vi "Veronica Maria - Simulador do Computador de Bordo.vi"() -> ()   [LabVIEW 2015]
uses:
  <vilib>/Instr/_visa.llb/VISA Configure Serial Port (Instr).vi
panel:
  out "Gráfico 2":u8(graph)
  out "Erro no diretório 2":errorcluster
  out "Arquivo Hexadecimal":refnum<file>
  out "Tempo da Varredura":dbl
  in  "DATA SEND":bool
  in  "DATA SEND":bool
  out "Erro serial":errorcluster
  out "Bytes Recebidos":u16
  out "Botao Selecionado":string
  out "Erros de entrada":errorcluster
  out "Erro no diretório":errorcluster
  out "Arquivo":refnum<file>
  out "Erros de envio entrada":errorcluster
  out "Saída de VISA Resource Name":refnum<visa-resource-name>
  out "PACOTE RECEBIDO":string
  out "frames":u8[][](array[numeric])
  out "frame enviado":u8[](array[numeric]) format="%x"
  in  "TURN OFF":bool
  in  "TURN ON":bool
  in  "DESLIGAR":bool
  in  "RESET":bool
  in  "DATA REQUEST":bool
  in  "diretório do arquivo":string="C:\\Testes\\"
  in  "bits de parada (8: 1 bit)":u8(ring)=10 items=["2.0"=20, "1.5"=15, "1.0"=10]
  in  "controle de fluxo (0: none)":u8(ring) items=["None", "XON/XOFF", "RTS/CTS", "XON/XOFF & RTS/CTS", "DTR/DSR", "XON/XOFF & DTS/DSR"]
  in  "taxa de transmissão (9600)":u16=9600
  in  "paridade (0: none)":u8(ring) items=["None", "Odd", "Even", "Mark", "Space"]
  in  "porta":refnum<visa-resource-name>
  in  "bits de dados(8)":u8=8 min=5 max=8 step=1
  # "Configurações \ndo \nSistema"
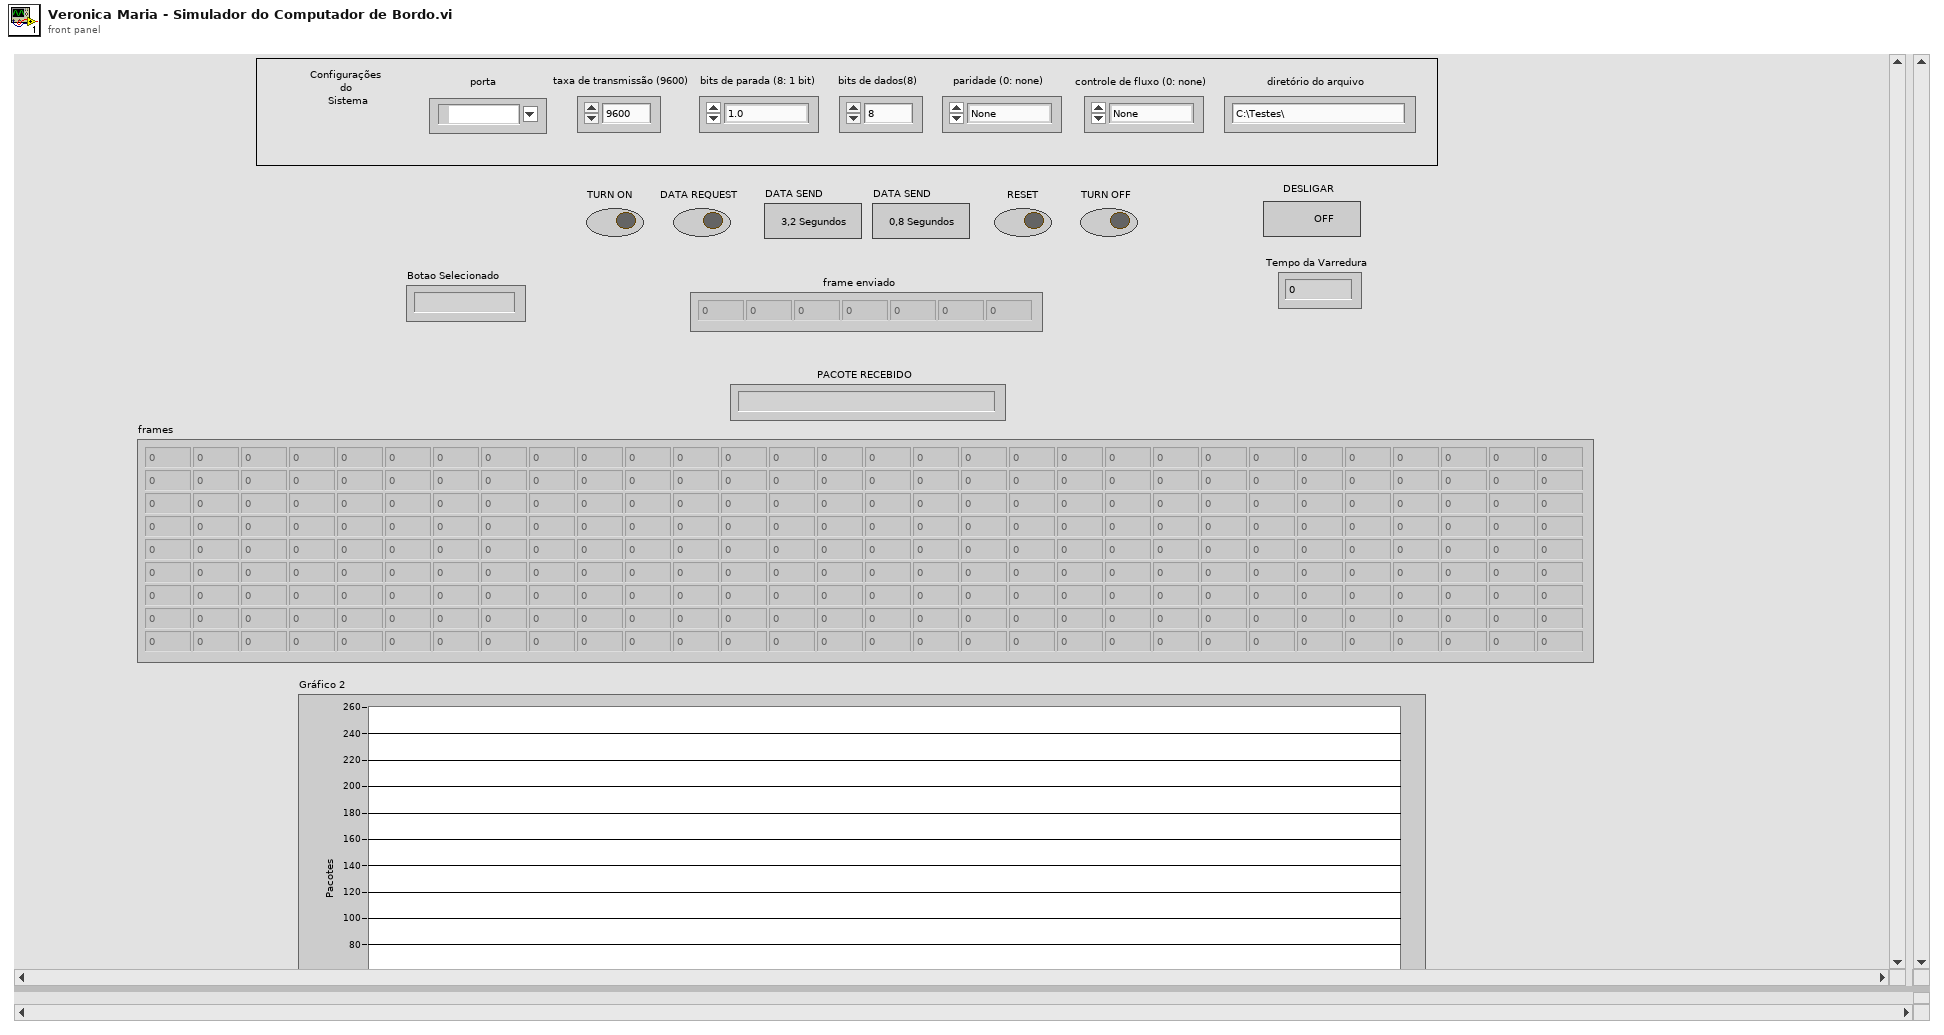
[diagram p1: front panel]
types:
  T1 = enum16{"open", "replace", "create", "open or create", "replace or create", "replace or create with confirmation"}
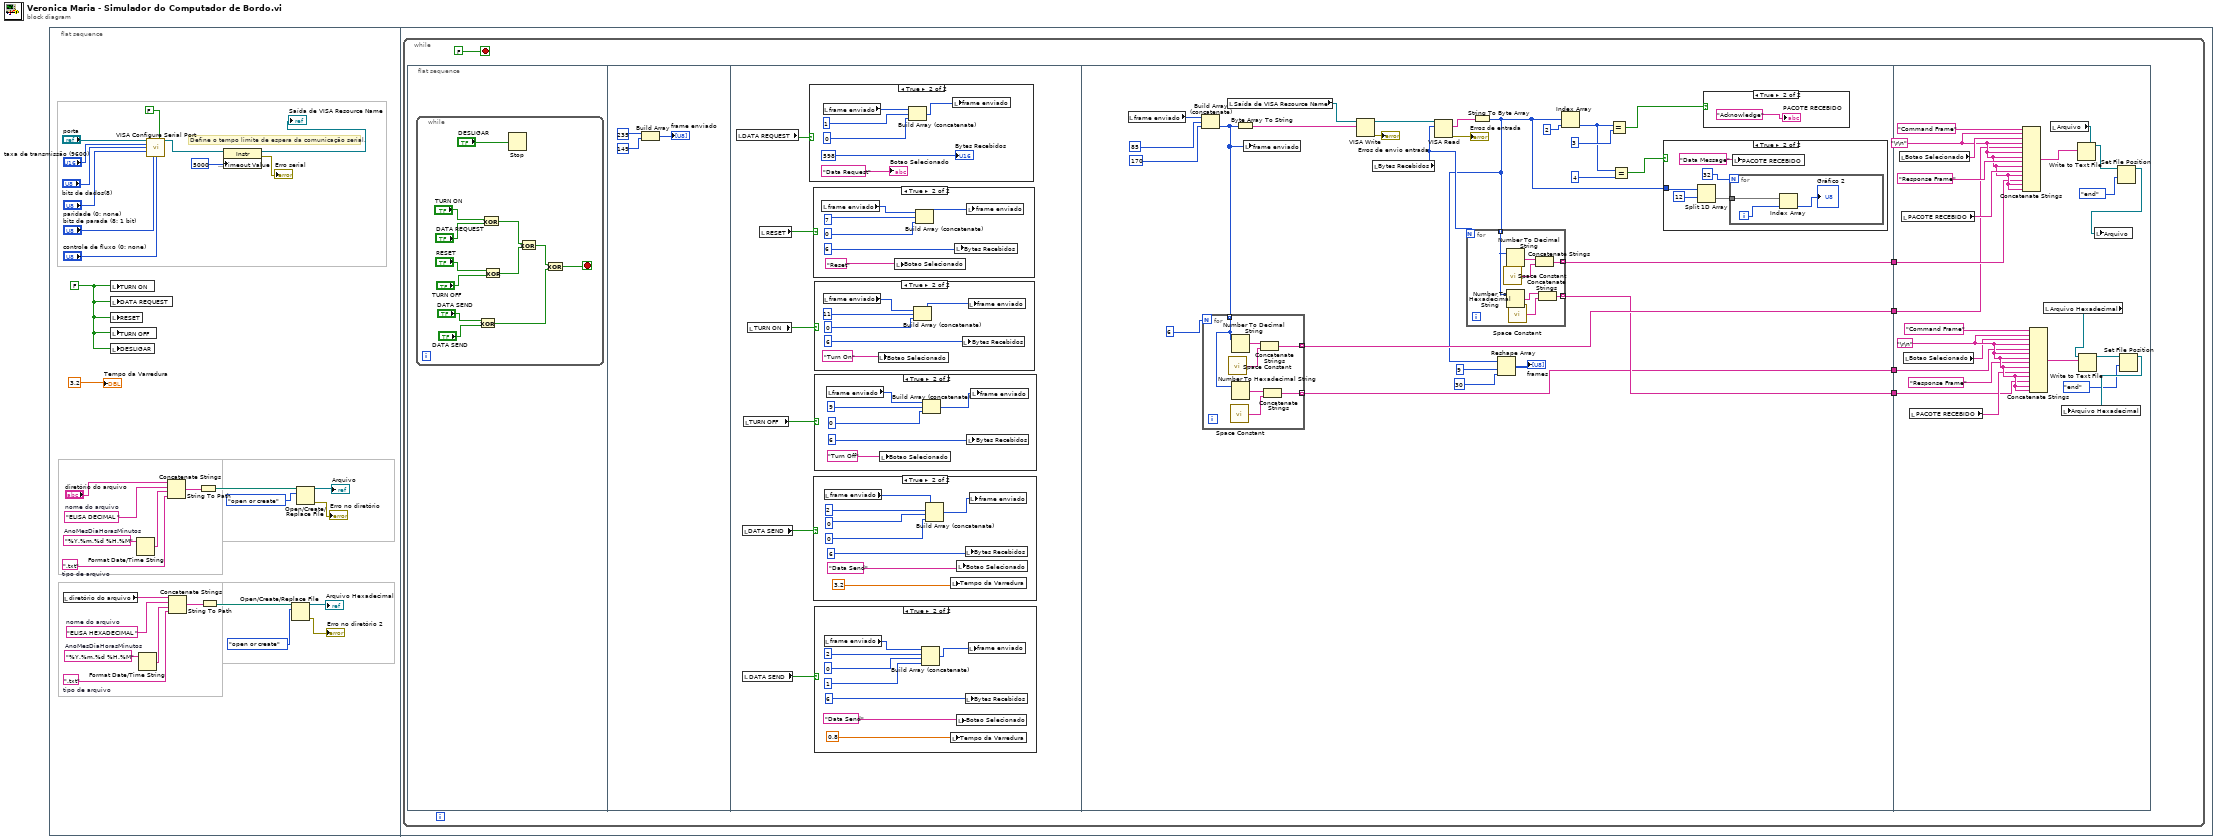
[diagram p0: block diagram]
diagram:
  n1 = flat-sequence {
    frame #0 {
      w10 = "%Y.%m.%d %H.%M"  # AnoMesDiaHorasMinutos
      w7 = ".txt"  # tipo de arquivo
      w9 = "ELISA HEXADECIMAL "  # nome do arquivo
      w16 = FALSE
      w26 = "%Y.%m.%d %H.%M"  # AnoMesDiaHorasMinutos
      w23 = ".txt"  # tipo de arquivo
      w25 = "ELISA DECIMAL "  # nome do arquivo
      # "Define o tempo limite de espera da comunicação serial."
      n2 = local read "diretório do arquivo"() -> (w1:string)
      n3 = local write "TURN ON"(w16) -> ()
      n4 = local write "DATA REQUEST"(w16) -> ()
      n5 = local write "RESET"(w16) -> ()
      n6 = local write "TURN OFF"(w16) -> ()
      n7 = local write "DESLIGAR"(w16) -> ()
      n8 = Format Date/Time String(time format string (%c)=w26) -> (date/time string=w24:string)  [unwired: 2 in]
      n9 = Format Date/Time String(time format string (%c)=w10) -> (date/time string=w8:string)  [unwired: 2 in]
      n10 = call-poly "VISA Configure Serial Port"("VISA resource name"="porta", "Enable Termination\nChar (T)"=FALSE, "baud rate (9600)"="taxa de transmissão (9600)", "data bits (8)"="bits de dados(8)", "parity (0:none)"="paridade (0: none)", "stop bits (10: 1 bit)"="bits de parada (8: 1 bit)", "flow control (0:none)"="controle de fluxo (0: none)") -> ("VISA resource name out"=w13:refnum<visa-resource-name>)  [unwired: 7 in, 1 out]
      n11 = Concatenate Strings("diretório do arquivo", w25, w24, w23) -> (w22:string)
      n12 = Concatenate Strings(w1, w9, w8, w7) -> (w6:string)
      n13 = String To Path(string=w22) -> (path=w21:path)
      n14 = String To Path(string=w6) -> (path=w3:path)
      n15 = property class="Instr"(reference=w13, "General Settings:Timeout Value"=u32 5000) -> (reference out=→"Saída de VISA Resource Name":refnum<visa-resource-name>, error out=→"Erro serial":errorcluster)  [unwired: 1 in]
      n16 = Open/Create/Replace File(file path (use dialog)=w3, operation (0:open)=T1."open or create") -> (refnum out=→"Arquivo Hexadecimal":refnum<file>, error out=→"Erro no diretório 2":errorcluster)  [unwired: 4 in, 1 out]
      n17 = Open/Create/Replace File(file path (use dialog)=w21, operation (0:open)=T1."open or create") -> (refnum out=→"Arquivo":refnum<file>, error out=→"Erro no diretório":errorcluster)  [unwired: 4 in, 1 out]
      "Tempo da Varredura" <- 3.2
    }
    frame #1 {
      n18 = while {
        stop <- FALSE stop-if-true
        n19 = flat-sequence {
          tunnel: [w109] -> w37
          tunnel: [w108] -> w36
          tunnel: [w100] -> w35
          tunnel: [w101] -> w34
          tunnel: w37 -> [w162]
          tunnel: w36 -> [w161]
          tunnel: w35 -> [w155]
          tunnel: w34 -> [w154]
          frame #0 {
            n20 = while {
              stop <- w39 stop-if-true
              n21 = Exclusive Or(1:"DATA SEND", 2:"DATA SEND") -> (0:w40:bool)
              n22 = Exclusive Or(1:"DATA REQUEST", 2:"TURN ON") -> (0:w43:bool)
              n23 = Exclusive Or(1:"TURN OFF", 2:"RESET") -> (0:w42:bool)
              n24 = Stop(stop? (T)="DESLIGAR") -> ()
              n25 = Exclusive Or(1:w42, 2:w43) -> (0:w41:bool)
              n26 = Exclusive Or(1:w40, 2:w41) -> (0:w39:bool)
            }
          }
          frame #1 {
            n27 = Build Array(235, 149) -> (→"frame enviado":i32[])
          }
          frame #2 {
            n28 = local read "DATA REQUEST"() -> (w59:bool)
            n29 = local read "DATA SEND"() -> (w55:bool)
            n30 = local read "DATA SEND"() -> (w54:bool)
            n31 = local read "TURN OFF"() -> (w56:bool)
            n32 = local read "TURN ON"() -> (w57:bool)
            n33 = local read "RESET"() -> (w58:bool)
            n34 = case shown="True" w59 {
              frame False {
              }
              frame True {
                n35 = local read "frame enviado"() -> (w99:u8[])
                n36 = Build Array (concatenate)(w99, 1, 0) -> (w95:i32[])
                n37 = local write "frame enviado"(w95) -> ()
                "Botao Selecionado" <- "Data Request"
                "Bytes Recebidos" <- 598
              }
            }
            n38 = case shown="True" w58 {
              frame False {
              }
              frame True {
                n39 = local read "frame enviado"() -> (w93:u8[])
                n40 = local write "Botao Selecionado"("Reset") -> ()
                n41 = Build Array (concatenate)(w93, 7, 0) -> (w90:i32[])
                n42 = local write "Bytes Recebidos"(6) -> ()
                n43 = local write "frame enviado"(w90) -> ()
              }
            }
            n44 = case shown="True" w55 {
              frame False {
              }
              frame True {
                n45 = local read "frame enviado"() -> (w75:u8[])
                n46 = Build Array (concatenate)(w75, 2, 0, 0) -> (w73:i32[])
                n47 = local write "Tempo da Varredura"(3.2) -> ()
                n48 = local write "Botao Selecionado"("Data Send") -> ()
                n49 = local write "Bytes Recebidos"(6) -> ()
                n50 = local write "frame enviado"(w73) -> ()
              }
            }
            n51 = case shown="True" w57 {
              frame False {
              }
              frame True {
                n52 = local read "frame enviado"() -> (w87:u8[])
                n53 = local write "Botao Selecionado"("Turn On") -> ()
                n54 = Build Array (concatenate)(w87, 11, 0) -> (w84:i32[])
                n55 = local write "Bytes Recebidos"(6) -> ()
                n56 = local write "frame enviado"(w84) -> ()
              }
            }
            n57 = case shown="True" w56 {
              frame False {
              }
              frame True {
                n58 = local read "frame enviado"() -> (w80:u8[])
                n59 = local write "Botao Selecionado"("Turn Off") -> ()
                n60 = Build Array (concatenate)(w80, 9, 0) -> (w78:i32[])
                n61 = local write "Bytes Recebidos"(6) -> ()
                n62 = local write "frame enviado"(w78) -> ()
              }
            }
            n63 = case shown="True" w54 {
              frame False {
              }
              frame True {
                n64 = local read "frame enviado"() -> (w67:u8[])
                n65 = Build Array (concatenate)(w67, 2, 0, 1) -> (w66:i32[])
                n66 = local write "Tempo da Varredura"(0.8) -> ()
                n67 = local write "Botao Selecionado"("Data Send") -> ()
                n68 = local write "Bytes Recebidos"(6) -> ()
                n69 = local write "frame enviado"(w66) -> ()
              }
            }
          }
          frame #3 {
            n70 = local read "frame enviado"() -> (w125:u8[])
            n71 = Build Array (concatenate)(w125, 85, 170) -> (w123:i32[])
            n72 = for {
              N: 6 -> [_]
              tunnel: w123 -> [w145] mode=indexing
              tunnel: [w147] -> w108 mode=indexing
              tunnel: [w142] -> w100 mode=indexing
              n73 = call <vilib>:"Space Constant.vi"() -> ("String"=w148:string)
              n74 = call <vilib>:"Space Constant.vi"() -> ("String"=w143:string)
              n75 = Number To Decimal String(number=w145) -> (decimal integer string=w146:string)  [unwired: 1 in]
              n76 = Number To Hexadecimal String(2:w145) -> (0:w144:string)  [unwired: 1 in]
              n77 = Concatenate Strings(w146, w148) -> (w147:string)
              n78 = Concatenate Strings(w144, w143) -> (w142:string)
            }
            n79 = local read "Saída de VISA Resource Name"() -> (w121:refnum<visa-resource-name>)
            n80 = Byte Array To String(unsigned byte array=w123) -> (string=w122:string)
            n81 = local write "frame enviado"(w123) -> ()
            n82 = VISA Write(VISA resource name=w121, write buffer=w122) -> (VISA resource name out=w119:refnum<visa-resource-name>, error out=→"Erros de envio entrada":errorcluster)  [unwired: 1 in, 1 out]
            n83 = local read "Bytes Recebidos"() -> (w110:u16)
            n84 = VISA Read(VISA resource name=w119, byte count=w110) -> (read buffer=w117:string, error out=→"Erros de entrada":errorcluster)  [unwired: 1 in, 2 out]
            n85 = String To Byte Array(string=w117) -> (unsigned byte array=w102:u8[])
            n86 = for {
              N: w110 -> [_]
              tunnel: w102 -> [w136] mode=indexing
              tunnel: [w140] -> w109 mode=indexing
              tunnel: [w135] -> w101 mode=indexing
              n87 = call <vilib>:"Space Constant.vi"() -> ("String"=w141:string)
              n88 = Number To Decimal String(number=w136) -> (decimal integer string=w139:string)  [unwired: 1 in]
              n89 = Number To Hexadecimal String(2:w136) -> (0:w138:string)  [unwired: 1 in]
              n90 = call <vilib>:"Space Constant.vi"() -> ("String"=w137:string)
              n91 = Concatenate Strings(w139, w141) -> (w140:string)
              n92 = Concatenate Strings(w138, w137) -> (w135:string)
            }
            n93 = Reshape Array(w102, u8 9, u8 30) -> (→"frames":u8[][])
            n94 = Index Array(array=w102, index=u8 2) -> (element=w107:u8)
            n95 = Equal?(x=w107, y=u8 3 ("index")) -> (x = y?=w111:bool)
            n96 = Equal?(x=w107, y=u8 4 ("index")) -> (x = y?=w105:bool)
            n97 = case shown="True" w105 {
              tunnel: w102 -> [_ w127]
              frame False {
              }
              frame True {
                n98 = Split 1D Array(array=w127, index=u8 12) -> (second subarray=w128:u8[])  [unwired: 1 out]
                n99 = for {
                  N: 32 -> [_]
                  tunnel: w128 -> [w133]
                  i -> [w132]
                  n100 = Index Array(array=w133, index=w132) -> (element=→"Gráfico 2":u8)
                }
                n101 = local write "PACOTE RECEBIDO"("Data Message") -> ()
              }
            }
            n102 = case shown="True" w111 {
              frame False {
              }
              frame True {
                "PACOTE RECEBIDO" <- "Acknowledge"
              }
            }
          }
          frame #4 {
            w159 = "\r\n"
            w163 = "\r\n"
            n103 = local read "Botao Selecionado"() -> (w166:string)
            n104 = local read "PACOTE RECEBIDO"() -> (w164:string)
            n105 = local read "Botao Selecionado"() -> (w158:string)
            n106 = local read "PACOTE RECEBIDO"() -> (w156:string)
            n107 = Concatenate Strings("Command Frame", w163, w166, w163, w161, w163, w163, "Response Frame", w163, w164, w163, w162, w163, w163) -> (w171:string)
            n108 = Concatenate Strings("Command Frame", w159, w158, w159, w155, w159, w159, "Response Frame", w159, w156, w159, w154, w159, w159) -> (w153:string)
            n109 = local read "Arquivo Hexadecimal"() -> (w149:refnum<file>)
            n110 = local read "Arquivo"() -> (w168:refnum<file>)
            n111 = Write to Text File(file (use dialog)=w168, text=w171) -> (refnum out=w170:refnum<file>)  [unwired: 2 in, 2 out]
            n112 = Write to Text File(file (use dialog)=w149, text=w153) -> (refnum out=w152:refnum<file>)  [unwired: 2 in, 2 out]
            n113 = Set File Position(refnum=w170, from (0:start)=enum16{"start", "end", "current"}."end") -> (refnum out=w167:refnum<file>)  [unwired: 2 in, 1 out]
            n114 = local write "Arquivo"(w167) -> ()
            n115 = Set File Position(refnum=w152, from (0:start)=enum16{"start", "end", "current"}."end") -> (refnum out=w151:refnum<file>)  [unwired: 2 in, 1 out]
            n116 = local write "Arquivo Hexadecimal"(w151) -> ()
          }
        }
      }
    }
  }
